vi "GeoData.vi"() -> ()   [LabVIEW 2017] (continued)
H1\n95924\t6057\tCedar ridge\tCA\tNevada County\tH1\n95728\t6057\tSoda springs\tCA\tNevada County\tH1\n95602\t6057\tAuburn\tCA\tNevada County\tH1\n95986\t6057\tWashington\tCA\tNevada County\tH1\n95712\t6057\tChicago park\tCA\tNevada County\tH1\n96161\t6057\tTruckee\tCA\tNevada County\tH1\n95949\t6057\tGrass valley\tCA\tNevada County\tH1\n95975\t6057\tRough and ready\tCA\tNevada County\tH1\n96160\t6057\tTruckee\tCA\tNevada County\tH1\n96111\t6057\tFloriston\tCA\tNevada County\tH1\n95945\t6057\tGrass valley\tCA\tNevada County\tH1\n95960\t6057\tNorth san juan\tCA\tNevada County\tH1\n95959\t6057\tNevada city\tCA\tNevada County\tH1\n90638\t6059\tLa mirada\tCA\tOrange County\tH1\n90680\t6059\tStanton\tCA\tOrange County\tH1\n92623\t6059\tIrvine\tCA\tOrange County\tH1\n92675\t6059\tSan juan capistrano\tCA\tOrange County\tH1\n92662\t6059\tNewport beach\tCA\tOrange County\tH1\n92693\t6059\tSan juan capistrano\tCA\tOrange County\tH1\n92694\t6059\tLadera ranch\tCA\tOrange County\tH1\n92825\t6059\tAnaheim\tCA\tOrange County\tH1\n92870\t6059\tPlacentia\tCA\tOrange County\tH1\n92811\t6059\tAtwood\tCA\tOrange County\tH1\n92616\t6059\tIrvine\tCA\tOrange County\tH1\n92702\t6059\tSanta ana\tCA\tOrange County\tH1\n92602\t6059\tIrvine\tCA\tOrange County\tH1\n92617\t6059\tIrvine\tCA\tOrange County\tH1\n92627\t6059\tCosta mesa\tCA\tOrange County\tH1\n92651\t6059\tLaguna beach\tCA\tOrange County\tH1\n92661\t6059\tNewport beach\tCA\tOrange County\tH1\n92637\t6059\tLaguna woods\tCA\tOrange County\tH1\n92688\t6059\tRancho santa margarita\tCA\tOrange County\tH1\n92654\t6059\tLaguna hills\tCA\tOrange County\tH1\n92782\t6059\tTustin\tCA\tOrange County\tH1\n92861\t6059\tVilla park\tCA\tOrange County\tH1\n92867\t6059\tOrange\tCA\tOrange County\tH1\n92886\t6059\tYorba linda\tCA\tOrange County\tH1\n92655\t6059\tMidway city\tCA\tOrange County\tH1\n92678\t6059\tTrabuco canyon\tCA\tOrange County\tH1\n90720\t6059\tLos alamitos\tCA\tOrange County\tH1\n90622\t6059\tBuena park\tCA\tOrange County\tH1\n92609\t6059\tEl toro\tCA\tOrange County\tH1\n92672\t6059\tSan clemente\tCA\tOrange County\tH1\n92630\t6059\tLake forest\tCA\tOrange County\tH1\n92648\t6059\tHuntington beach\tCA\tOrange County\tH1\n92692\t6059\tMission viejo\tCA\tOrange County\tH1\n92701\t6059\tSanta ana\tCA\tOrange County\tH1\n92801\t6059\tAnaheim\tCA\tOrange County\tH1\n92804\t6059\tAnaheim\tCA\tOrange County\tH1\n92808\t6059\tAnaheim\tCA\tOrange County\tH1\n92821\t6059\tBrea\tCA\tOrange County\tH1\n92831\t6059\tFullerton\tCA\tOrange County\tH1\n92840\t6059\tGarden grove\tCA\tOrange County\tH1\n92803\t6059\tAnaheim\tCA\tOrange County\tH1\n92868\t6059\tOrange\tCA\tOrange County\tH1\n92822\t6059\tBrea\tCA\tOrange County\tH1\n92863\t6059\tOrange\tCA\tOrange County\tH1\n90721\t6059\tLos alamitos\tCA\tOrange County\tH1\n92846\t6059\tGarden grove\tCA\tOrange County\tH1\n92698\t6059\tAliso viejo\tCA\tOrange County\tH1\n92864\t6059\tOrange\tCA\tOrange County\tH1\n90624\t6059\tBuena park\tCA\tOrange County\tH1\n90740\t6059\tSeal beach\tCA\tOrange County\tH1\n90621\t6059\tBuena park\tCA\tOrange County\tH1\n90620\t6059\tBuena park\tCA\tOrange County\tH1\n92603\t6059\tIrvine\tCA\tOrange County\tH1\n92649\t6059\tHuntington beach\tCA\tOrange County\tH1\n92663\t6059\tNewport beach\tCA\tOrange County\tH1\n92657\t6059\tNewport coast\tCA\tOrange County\tH1\n92677\t6059\tLaguna niguel\tCA\tOrange County\tH1\n92691\t6059\tMission viejo\tCA\tOrange County\tH1\n92780\t6059\tTustin\tCA\tOrange County\tH1\n92805\t6059\tAnaheim\tCA\tOrange County\tH1\n92807\t6059\tAnaheim\tCA\tOrange County\tH1\n92704\t6059\tSanta ana\tCA\tOrange County\tH1\n92706\t6059\tSanta ana\tCA\tOrange County\tH1\n92806\t6059\tAnaheim\tCA\tOrange County\tH1\n92841\t6059\tGarden grove\tCA\tOrange County\tH1\n92843\t6059\tGarden grove\tCA\tOrange County\tH1\n92711\t6059\tSanta ana\tCA\tOrange County\tH1\n92815\t6059\tAnaheim\tCA\tOrange County\tH1\n92869\t6059\tOrange\tCA\tOrange County\tH1\n90633\t6059\tLa habra\tCA\tOrange County\tH1\n90742\t6059\tSunset beach\tCA\tOrange County\tH1\n92857\t6059\tOrange\tCA\tOrange County\tH1\n90743\t6059\tSurfside\tCA\tOrange County\tH1\n90815\t6059\tLong beach\tCA\tOrange County\tH1\n92604\t6059\tIrvine\tCA\tOrange County\tH1\n92612\t6059\tIrvine\tCA\tOrange County\tH1\n92618\t6059\tIrvine\tCA\tOrange County\tH1\n92620\t6059\tIrvine\tCA\tOrange County\tH1\n92625\t6059\tCorona del mar\tCA\tOrange County\tH1\n92614\t6059\tIrvine\tCA\tOrange County\tH1\n92629\t6059\tDana point\tCA\tOrange County\tH1\n92697\t6059\tIrvine\tCA\tOrange County\tH1\n92802\t6059\tAnaheim\tCA\tOrange County\tH1\n92823\t6059\tBrea\tCA\tOrange County\tH1\n92844\t6059\tGarden grove\tCA\tOrange County\tH1\n92866\t6059\tOrange\tCA\tOrange County\tH1\n92619\t6059\tIrvine\tCA\tOrange County\tH1\n92676\t6059\tSilverado\tCA\tOrange County\tH1\n92684\t6059\tWestminster\tCA\tOrange County\tH1\n92871\t6059\tPlacentia\tCA\tOrange County\tH1\n92816\t6059\tAnaheim\tCA\tOrange County\tH1\n90631\t6059\tLa habra\tCA\tOrange County\tH1\n92610\t6059\tFoothill ranch\tCA\tOrange County\tH1\n92626\t6059\tCosta mesa\tCA\tOrange County\tH1\n92624\t6059\tCapistrano beach\tCA\tOrange County\tH1\n92647\t6059\tHuntington beach\tCA\tOrange County\tH1\n92673\t6059\tSan clemente\tCA\tOrange County\tH1\n92685\t6059\tWestminster\tCA\tOrange County\tH1\n92707\t6059\tSanta ana\tCA\tOrange County\tH1\n92708\t6059\tFountain valley\tCA\tOrange County\tH1\n92781\t6059\tTustin\tCA\tOrange County\tH1\n92812\t6059\tAnaheim\tCA\tOrange County\tH1\n92865\t6059\tOrange\tCA\tOrange County\tH1\n92887\t6059\tYorba linda\tCA\tOrange County\tH1\n92817\t6059\tAnaheim\tCA\tOrange County\tH1\n92834\t6059\tFullerton\tCA\tOrange County\tH1\n92838\t6059\tFullerton\tCA\tOrange County\tH1\n92607\t6059\tLaguna niguel\tCA\tOrange County\tH1\n92859\t6059\tOrange\tCA\tOrange County\tH1\n90632\t6059\tLa habra\tCA\tOrange County\tH1\n92836\t6059\tFullerton\tCA\tOrange County\tH1\n90623\t6059\tLa palma\tCA\tOrange County\tH1\n92653\t6059\tLaguna hills\tCA\tOrange County\tH1\n92646\t6059\tHuntington beach\tCA\tOrange County\tH1\n92650\t6059\tEast irvine\tCA\tOrange County\tH1\n92679\t6059\tTrabuco canyon\tCA\tOrange County\tH1\n92703\t6059\tSanta ana\tCA\tOrange County\tH1\n92705\t6059\tSanta ana\tCA\tOrange County\tH1\n92845\t6059\tGarden grove\tCA\tOrange County\tH1\n92837\t6059\tFullerton\tCA\tOrange County\tH1\n92832\t6059\tFullerton\tCA\tOrange County\tH1\n92652\t6059\tLaguna beach\tCA\tOrange County\tH1\n92799\t6059\tSanta ana\tCA\tOrange County\tH1\n92728\t6059\tFountain valley\tCA\tOrange County\tH1\n92735\t6059\tSanta ana\tCA\tOrange County\tH1\n92814\t6059\tAnaheim\tCA\tOrange County\tH1\n92862\t6059\tOrange\tCA\tOrange County\tH1\n90808\t6059\tLong beach\tCA\tOrange County\tH1\n90630\t6059\tCypress\tCA\tOrange County\tH1\n92605\t6059\tHuntington beach\tCA\tOrange County\tH1\n92606\t6059\tIrvine\tCA\tOrange County\tH1\n92656\t6059\tAliso viejo\tCA\tOrange County\tH1\n92660\t6059\tNewport beach\tCA\tOrange County\tH1\n92674\t6059\tSan clemente\tCA\tOrange County\tH1\n92683\t6059\tWestminster\tCA\tOrange County\tH1\n92658\t6059\tNewport beach\tCA\tOrange County\tH1\n92690\t6059\tMission viejo\tCA\tOrange County\tH1\n92628\t6059\tCosta mesa\tCA\tOrange County\tH1\n92835\t6059\tFullerton\tCA\tOrange County\tH1\n92842\t6059\tGarden grove\tCA\tOrange County\tH1\n92856\t6059\tOrange\tCA\tOrange County\tH1\n92833\t6059\tFullerton\tCA\tOrange County\tH1\n92809\t6059\tAnaheim\tCA\tOrange County\tH1\n92615\t6059\tHuntington beach\tCA\tOrange County\tH1\n92659\t6059\tNewport beach\tCA\tOrange County\tH1\n92885\t6059\tYorba linda\tCA\tOrange County\tH1\n92899\t6059\tAnaheim\tCA\tOrange County\tH1\n95631\t6061\tForesthill\tCA\tPlacer County\tH1\n95722\t6061\tMeadow vista\tCA\tPlacer County\tH1\n95650\t6061\tLoomis\tCA\tPlacer County\tH1\n95661\t6061\tRoseville\tCA\tPlacer County\tH1\n95765\t6061\tRocklin\tCA\tPlacer County\tH1\n96146\t6061\tOlympic valley\tCA\tPlacer County\tH1\n96145\t6061\tTahoe city\tCA\tPlacer County\tH1\n96148\t6061\tTahoe vista\tCA\tPlacer County\tH1\n95701\t6061\tAlta\tCA\tPlacer County\tH1\n95703\t6061\tApplegate\tCA\tPlacer County\tH1\n96141\t6061\tHomewood\tCA\tPlacer County\tH1\n95602\t6061\tAuburn\tCA\tPlacer County\tH1\n95663\t6061\tPenryn\tCA\tPlacer County\tH1\n96143\t6061\tKings beach\tCA\tPlacer County\tH1\n96161\t6061\tTruckee\tCA\tPlacer County\tH1\n95648\t6061\tLincoln\tCA\tPlacer County\tH1\n95626\t6061\tElverta\tCA\tPlacer County\tH1\n95658\t6061\tNewcastle\tCA\tPlacer County\tH1\n95746\t6061\tGranite bay\tCA\tPlacer County\tH1\n95747\t6061\tRoseville\tCA\tPlacer County\tH1\n95713\t6061\tColfax\tCA\tPlacer County\tH1\n95714\t6061\tDutch flat\tCA\tPlacer County\tH1\n95715\t6061\tEmigrant gap\tCA\tPlacer County\tH1\n95717\t6061\tGold run\tCA\tPlacer County\tH1\n95681\t6061\tSheridan\tCA\tPlacer County\tH1\n95610\t6061\tCitrus heights\tCA\tPlacer County\tH1\n95603\t6061\tAuburn\tCA\tPlacer County\tH1\n95604\t6061\tAuburn\tCA\tPlacer County\tH1\n95678\t6061\tRoseville\tCA\tPlacer County\tH1\n95677\t6061\tRocklin\tCA\tPlacer County\tH1\n96142\t6061\tTahoma\tCA\tPlacer County\tH1\n95668\t6061\tPleasant grove\tCA\tPlacer County\tH1\n96140\t6061\tCarnelian bay\tCA\tPlacer County\tH1\n95736\t6061\tWeimar\tCA\tPlacer County\tH1\n95983\t6063\tTaylorsville\tCA\tPlumas County\tH1\n96105\t6063\tChilcoot\tCA\tPlumas County\tH1\n96122\t6063\tPortola\tCA\tPlumas County\tH1\n95971\t6063\tQuincy\tCA\tPlumas County\tH1\n96135\t6063\tVinton\tCA\tPlumas County\tH1\n95956\t6063\tMeadow valley\tCA\tPlumas County\tH1\n95947\t6063\tGreenville\tCA\tPlumas County\tH1\n95980\t6063\tStorrie\tCA\tPlumas County\tH1\n95915\t6063\tBelden\tCA\tPlumas County\tH1\n95981\t6063\tStrawberry valley\tCA\tPlumas County\tH1\n95930\t6063\tClipper mills\tCA\tPlumas County\tH1\n95984\t6063\tTwain\tCA\tPlumas County\tH1\n96020\t6063\tChester\tCA\tPlumas County\tH1\n96137\t6063\tWestwood\tCA\tPlumas County\tH1\n96129\t6063\tBeckwourth\tCA\tPlumas County\tH1\n95934\t6063\tCrescent mills\tCA\tPlumas County\tH1\n96106\t6063\tClio\tCA\tPlumas County\tH1\n95923\t6063\tCanyon dam\tCA\tPlumas County\tH1\n96103\t6063\tBlairsden graeagle\tCA\tPlumas County\tH1\n92373\t6065\tRedlands\tCA\tRiverside County\tH1\n92595\t6065\tWildomar\tCA\tRiverside County\tH1\n92518\t6065\tMarch air reserve base\tCA\tRiverside County\tH1\n92530\t6065\tLake elsinore\tCA\tRiverside County\tH1\n92548\t6065\tHomeland\tCA\tRiverside County\tH1\n92508\t6065\tRiverside\tCA\tRiverside County\tH1\n92552\t6065\tMoreno valley\tCA\tRiverside County\tH1\n92262\t6065\tPalm springs\tCA\tRiverside County\tH1\n92522\t6065\tRiverside\tCA\tRiverside County\tH1\n92220\t6065\tBanning\tCA\tRiverside County\tH1\n92591\t6065\tTemecula\tCA\tRiverside County\tH1\n92582\t6065\tSan jacinto\tCA\tRiverside County\tH1\n92531\t6065\tLake elsinore\tCA\tRiverside County\tH1\n92562\t6065\tMurrieta\tCA\tRiverside County\tH1\n92551\t6065\tMoreno valley\tCA\tRiverside County\tH1\n92581\t6065\tSan jacinto\tCA\tRiverside County\tH1\n92203\t6065\tIndio\tCA\tRiverside County\tH1\n92211\t6065\tPalm desert\tCA\tRiverside County\tH1\n92590\t6065\tTemecula\tCA\tRiverside County\tH1\n92592\t6065\tTemecula\tCA\tRiverside County\tH1\n92571\t6065\tPerris\tCA\tRiverside County\tH1\n92507\t6065\tRiverside\tCA\tRiverside County\tH1\n92532\t6065\tLake elsinore\tCA\tRiverside County\tH1\n92539\t6065\tAnza\tCA\tRiverside County\tH1\n92563\t6065\tMurrieta\tCA\tRiverside County\tH1\n92567\t6065\tNuevo\tCA\tRiverside County\tH1\n92240\t6065\tDesert hot springs\tCA\tRiverside County\tH1\n92234\t6065\tCathedral city\tCA\tRiverside County\tH1\n92241\t6065\tDesert hot springs\tCA\tRiverside County\tH1\n92883\t6065\tCorona\tCA\tRiverside County\tH1\n92513\t6065\tRiverside\tCA\tRiverside County\tH1\n92248\t6065\tLa quinta\tCA\tRiverside County\tH1\n92517\t6065\tRiverside\tCA\tRiverside County\tH1\n92226\t6065\tBlythe\tCA\tRiverside County\tH1\n92564\t6065\tMurrieta\tCA\tRiverside County\tH1\n92399\t6065\tYucaipa\tCA\tRiverside County\tH1\n92596\t6065\tWinchester\tCA\tRiverside County\tH1\n92586\t6065\tMenifee\tCA\tRiverside County\tH1\n91708\t6065\tChino\tCA\tRiverside County\tH1\n92509\t6065\tJurupa valley\tCA\tRiverside County\tH1\n92519\t6065\tRiverside\tCA\tRiverside County\tH1\n92505\t6065\tRiverside\tCA\tRiverside County\tH1\n92553\t6065\tMoreno valley\tCA\tRiverside County\tH1\n92253\t6065\tLa quinta\tCA\tRiverside County\tH1\n92236\t6065\tCoachella\tCA\tRiverside County\tH1\n92282\t6065\tWhitewater\tCA\tRiverside County\tH1\n92860\t6065\tNorco\tCA\tRiverside County\tH1\n92882\t6065\tCorona\tCA\tRiverside County\tH1\n92514\t6065\tRiverside\tCA\tRiverside County\tH1\n92247\t6065\tLa quinta\tCA\tRiverside County\tH1\n92028\t6065\tFallbrook\tCA\tRiverside County\tH1\n92201\t6065\tIndio\tCA\tRiverside County\tH1\n92585\t6065\tMenifee\tCA\tRiverside County\tH1\n92593\t6065\tTemecula\tCA\tRiverside County\tH1\n91752\t6065\tMira loma\tCA\tRiverside County\tH1\n92555\t6065\tMoreno valley\tCA\tRiverside County\tH1\n92546\t6065\tHemet\tCA\tRiverside County\tH1\n92223\t6065\tBeaumont\tCA\tRiverside County\tH1\n92254\t6065\tMecca\tCA\tRiverside County\tH1\n92230\t6065\tCabazon\tCA\tRiverside County\tH1\n92263\t6065\tPalm springs\tCA\tRiverside County\tH1\n92255\t6065\tPalm desert\tCA\tRiverside County\tH1\n92589\t6065\tTemecula\tCA\tRiverside County\tH1\n92239\t6065\tDesert center\tCA\tRiverside County\tH1\n92210\t6065\tIndian wells\tCA\tRiverside County\tH1\n92320\t6065\tCalimesa\tCA\tRiverside County\tH1\n92584\t6065\tMenifee\tCA\tRiverside County\tH1\n92587\t6065\tMenifee\tCA\tRiverside County\tH1\n92544\t6065\tHemet\tCA\tRiverside County\tH1\n92543\t6065\tHemet\tCA\tRiverside County\tH1\n92503\t6065\tRiverside\tCA\tRiverside County\tH1\n92261\t6065\tPalm desert\tCA\tRiverside County\tH1\n92274\t6065\tThermal\tCA\tRiverside County\tH1\n92202\t6065\tIndio\tCA\tRiverside County\tH1\n92556\t6065\tMoreno valley\tCA\tRiverside County\tH1\n92549\t6065\tIdyllwild\tCA\tRiverside County\tH1\n92258\t6065\tNorth palm springs\tCA\tRiverside County\tH1\n92521\t6065\tRiverside\tCA\tRiverside County\tH1\n92599\t6065\tPerris\tCA\tRiverside County\tH1\n92572\t6065\tPerris\tCA\tRiverside County\tH1\n91762\t6065\tOntario\tCA\tRiverside County\tH1\n92506\t6065\tRiverside\tCA\tRiverside County\tH1\n92504\t6065\tRiverside\tCA\tRiverside County\tH1\n92545\t6065\tHemet\tCA\tRiverside County\tH1\n92536\t6065\tAguanga\tCA\tRiverside County\tH1\n92561\t6065\tMountain center\tCA\tRiverside County\tH1\n92260\t6065\tPalm desert\tCA\tRiverside County\tH1\n92225\t6065\tBlythe\tCA\tRiverside County\tH1\n92270\t6065\tRancho mirage\tCA\tRiverside County\tH1\n92878\t6065\tCorona\tCA\tRiverside County\tH1\n92877\t6065\tCorona\tCA\tRiverside County\tH1\n92502\t6065\tRiverside\tCA\tRiverside County\tH1\n92324\t6065\tColton\tCA\tRiverside County\tH1\n92570\t6065\tPerris\tCA\tRiverside County\tH1\n92583\t6065\tSan jacinto\tCA\tRiverside County\tH1\n92557\t6065\tMoreno valley\tCA\tRiverside County\tH1\n92501\t6065\tRiverside\tCA\tRiverside County\tH1\n92516\t6065\tRiverside\tCA\tRiverside County\tH1\n92264\t6065\tPalm springs\tCA\tRiverside County\tH1\n92235\t6065\tCathedral city\tCA\tRiverside County\tH1\n92276\t6065\tThousand palms\tCA\tRiverside County\tH1\n92879\t6065\tCorona\tCA\tRiverside County\tH1\n92880\t6065\tCorona\tCA\tRiverside County\tH1\n92881\t6065\tCorona\tCA\tRiverside County\tH1\n95630\t6067\tFolsom\tCA\tSacramento County\tH1\n95683\t6067\tSloughhouse\tCA\tSacramento County\tH1\n95820\t6067\tSacramento\tCA\tSacramento County\tH1\n95864\t6067\tSacramento\tCA\tSacramento County\tH1\n95826\t6067\tSacramento\tCA\tSacramento County\tH1\n95690\t6067\tWalnut grove\tCA\tSacramento County\tH1\n95661\t6067\tRoseville\tCA\tSacramento County\tH1\n95611\t6067\tCitrus heights\tCA\tSacramento County\tH1\n95812\t6067\tSacramento\tCA\tSacramento County\tH1\n95823\t6067\tSacramento\tCA\tSacramento County\tH1\n95835\t6067\tSacramento\tCA\tSacramento County\tH1\n95671\t6067\tRepresa\tCA\tSacramento County\tH1\n95662\t6067\tOrangevale\tCA\tSacramento County\tH1\n95814\t6067\tSacramento\tCA\tSacramento County\tH1\n95818\t6067\tSacramento\tCA\tSacramento County\tH1\n95838\t6067\tSacramento\tCA\tSacramento County\tH1\n95831\t6067\tSacramento\tCA\tSacramento County\tH1\n95833\t6067\tSacramento\tCA\tSacramento County\tH1\n95759\t6067\tElk grove\tCA\tSacramento County\tH1\n95853\t6067\tSacramento\tCA\tSacramento County\tH1\n95628\t6067\tFair oaks\tCA\tSacramento County\tH1\n95621\t6067\tCitrus heights\tCA\tSacramento County\tH1\n95741\t6067\tRancho cordova\tCA\tSacramento County\tH1\n95819\t6067\tSacramento\tCA\tSacramento County\tH1\n95830\t6067\tSacramento\tCA\tSacramento County\tH1\n95840\t6067\tSacramento\tCA\tSacramento County\tH1\n95626\t6067\tElverta\tCA\tSacramento County\tH1\n95673\t6067\tRio linda\tCA\tSacramento County\tH1\n95670\t6067\tRancho cordova\tCA\tSacramento County\tH1\n95652\t6067\tMcclellan\tCA\tSacramento County\tH1\n95660\t6067\tNorth highlands\tCA\tSacramento County\tH1\n95757\t6067\tElk grove\tCA\tSacramento County\tH1\n95815\t6067\tSacramento\tCA\tSacramento County\tH1\n95822\t6067\tSacramento\tCA\tSacramento County\tH1\n95693\t6067\tWilton\tCA\tSacramento County\tH1\n95828\t6067\tSacramento\tCA\tSacramento County\tH1\n95834\t6067\tSacramento\tCA\tSacramento County\tH1\n95860\t6067\tSacramento\tCA\tSacramento County\tH1\n95842\t6067\tSacramento\tCA\tSacramento County\tH1\n95813\t6067\tSacramento\tCA\tSacramento County\tH1\n95867\t6067\tSacramento\tCA\tSacramento County\tH1\n95836\t6067\tSacramento\tCA\tSacramento County\tH1\n94571\t6067\tRio vista\tCA\tSacramento County\tH1\n95624\t6067\tElk grove\tCA\tSacramento County\tH1\n95632\t6067\tGalt\tCA\tSacramento County\tH1\n95825\t6067\tSacramento\tCA\tSacramento County\tH1\n95821\t6067\tSacramento\tCA\tSacramento County\tH1\n95841\t6067\tSacramento\tCA\tSacramento County\tH1\n95827\t6067\tSacramento\tCA\tSacramento County\tH1\n95843\t6067\tAntelope\tCA\tSacramento County\tH1\n95837\t6067\tSacramento\tCA\tSacramento County\tH1\n95866\t6067\tSacramento\tCA\tSacramento County\tH1\n95894\t6067\tSacramento\tCA\tSacramento County\tH1\n95816\t6067\tSacramento\tCA\tSacramento County\tH1\n95824\t6067\tSacramento\tCA\tSacramento County\tH1\n95829\t6067\tSacramento\tCA\tSacramento County\tH1\n95832\t6067\tSacramento\tCA\tSacramento County\tH1\n95638\t6067\tHerald\tCA\tSacramento County\tH1\n95641\t6067\tIsleton\tCA\tSacramento County\tH1\n95851\t6067\tSacramento\tCA\tSacramento County\tH1\n95615\t6067\tCourtland\tCA\tSacramento County\tH1\n95608\t6067\tCarmichael\tCA\tSacramento County\tH1\n95610\t6067\tCitrus heights\tCA\tSacramento County\tH1\n95609\t6067\tCarmichael\tCA\tSacramento County\tH1\n95655\t6067\tMather\tCA\tSacramento County\tH1\n95758\t6067\tElk grove\tCA\tSacramento County\tH1\n95811\t6067\tSacramento\tCA\tSacramento County\tH1\n95678\t6067\tRoseville\tCA\tSacramento County\tH1\n95817\t6067\tSacramento\tCA\tSacramento County\tH1\n95742\t6067\tRancho cordova\tCA\tSacramento County\tH1\n95852\t6067\tSacramento\tCA\tSacramento County\tH1\n95763\t6067\tFolsom\tCA\tSacramento County\tH1\n95865\t6067\tSacramento\tCA\tSacramento County\tH1\n95639\t6067\tHood\tCA\tSacramento County\tH1\n95680\t6067\tRyde\tCA\tSacramento County\tH1\n95004\t6069\tAromas\tCA\tSan Benito County\tH1\n93925\t6069\tChualar\tCA\tSan Benito County\tH1\n95043\t6069\tPaicines\tCA\tSan Benito County\tH1\n95024\t6069\tHollister\tCA\tSan Benito County\tH1\n95075\t6069\tTres pinos\tCA\tSan Benito County\tH1\n95045\t6069\tSan juan bautista\tCA\tSan Benito County\tH1\n95023\t6069\tHollister\tCA\tSan Benito County\tH1\n92344\t6071\tHesperia\tCA\tSan Bernardino County\tH1\n92345\t6071\tHesperia\tCA\tSan Bernardino County\tH1\n92373\t6071\tRedlands\tCA\tSan Bernardino County\tH1\n92356\t6071\tLucerne valley\tCA\tSan Bernardino County\tH1\n92394\t6071\tVictorville\tCA\tSan Bernardino County\tH1\n92335\t6071\tFontana\tCA\tSan Bernardino County\tH1\n92404\t6071\tSan bernardino\tCA\tSan Bernardino County\tH1\n91730\t6071\tRancho cucamonga\tCA\tSan Bernardino County\tH1\n91764\t6071\tOntario\tCA\tSan Bernardino County\tH1\n92372\t6071\tPinon hills\tCA\tSan Bernardino County\tH1\n91785\t6071\tUpland\tCA\tSan Bernardino County\tH1\n92305\t6071\tAngelus oaks\tCA\tSan Bernardino County\tH1\n92317\t6071\tBlue jay\tCA\tSan Bernardino County\tH1\n91759\t6071\tMt baldy\tCA\tSan Bernardino County\tH1\n92352\t6071\tLake arrowhead\tCA\tSan Bernardino County\tH1\n92402\t6071\tSan bernardino\tCA\tSan Bernardino County\tH1\n91784\t6071\tUpland\tCA\tSan Bernardino County\tH1\n91763\t6071\tMontclair\tCA\tSan Bernardino County\tH1\n92423\t6071\tSan bernardino\tCA\tSan Bernardino County\tH1\n92277\t6071\tTwentynine palms\tCA\tSan Bernardino County\tH1\n92284\t6071\tYucca valley\tCA\tSan Bernardino County\tH1\n92285\t6071\tLanders\tCA\tSan Bernardino County\tH1\n92332\t6071\tEssex\tCA\tSan Bernardino County\tH1\n92366\t6071\tMountain pass\tCA\tSan Bernardino County\tH1\n92312\t6071\tBarstow\tCA\tSan Bernardino County\tH1\n92369\t6071\tPatton\tCA\tSan Bernardino County\tH1\n92418\t6071\tSan bernardino\tCA\tSan Bernardino County\tH1\n93555\t6071\tRidgecrest\tCA\tSan Bernardino County\tH1\n92313\t6071\tGrand terrace\tCA\tSan Bernardino County\tH1\n92316\t6071\tBloomington\tCA\tSan Bernardino County\tH1\n92365\t6071\tNewberry springs\tCA\tSan Bernardino County\tH1\n92368\t6071\tOro grande\tCA\tSan Bernardino County\tH1\n92342\t6071\tHelendale\tCA\tSan Bernardino County\tH1\n92406\t6071\tSan bernardino\tCA\tSan Bernardino County\tH1\n91709\t6071\tChino hills\tCA\tSan Bernardino County\tH1\n92364\t6071\tNipton\tCA\tSan Bernardino County\tH1\n92340\t6071\tHesperia\tCA\tSan Bernardino County\tH1\n92315\t6071\tBig bear lake\tCA\tSan Bernardino County\tH1\n92393\t6071\tVictorville\tCA\tSan Bernardino County\tH1\n92382\t6071\tRunning springs\tCA\tSan Bernardino County\tH1\n92304\t6071\tAmboy\tCA\tSan Bernardino County\tH1\n92403\t6071\tSan bernardino\tCA\tSan Bernardino County\tH1\n92318\t6071\tBryn mawr\tCA\tSan Bernardino County\tH1\n92399\t6071\tYucaipa\tCA\tSan Bernardino County\tH1\n91710\t6071\tChino\tCA\tSan Bernardino County\tH1\n91737\t6071\tRancho cucamonga\tCA\tSan Bernardino County\tH1\n91708\t6071\tChino\tCA\tSan Bernardino County\tH1\n92509\t6071\tJurupa valley\tCA\tSan Bernardino County\tH1\n92256\t6071\tMorongo valley\tCA\tSan Bernardino County\tH1\n92386\t6071\tSugarloaf\tCA\tSan Bernardino County\tH1\n92278\t6071\tTwentynine palms\tCA\tSan Bernardino County\tH1\n93562\t6071\tTrona\tCA\tSan Bernardino County\tH1\n92392\t6071\tVictorville\tCA\tSan Bernardino County\tH1\n92374\t6071\tRedlands\tCA\tSan Bernardino County\tH1\n92363\t6071\tNeedles\tCA\tSan Bernardino County\tH1\n92310\t6071\tFort irwin\tCA\tSan Bernardino County\tH1\n92407\t6071\tSan bernardino\tCA\tSan Bernardino County\tH1\n91701\t6071\tRancho cucamonga\tCA\tSan Bernardino County\tH1\n91761\t6071\tOntario\tCA\tSan Bernardino County\tH1\n91729\t6071\tRancho cucamonga\tCA\tSan Bernardino County\tH1\n91752\t6071\tMira loma\tCA\tSan Bernardino County\tH1\n92223\t6071\tBeaumont\tCA\tSan Bernardino County\tH1\n92301\t6071\tAdelanto\tCA\tSan Bernardino County\tH1\n92329\t6071\tPhelan\tCA\tSan Bernardino County\tH1\n92401\t6071\tSan bernardino\tCA\tSan Bernardino County\tH1\n92391\t6071\tTwin peaks\tCA\tSan Bernardino County\tH1\n92350\t6071\tLoma linda\tCA\tSan Bernardino County\tH1\n92331\t6071\tFontana\tCA\tSan Bernardino County\tH1\n92280\t6071\tVidal\tCA\tSan Bernardino County\tH1\n92322\t6071\tCedarpines park\tCA\tSan Bernardino County\tH1\n92341\t6071\tGreen valley lake\tCA\tSan Bernardino County\tH1\n92267\t6071\tParker dam\tCA\tSan Bernardino County\tH1\n93516\t6071\tBoron\tCA\tSan Bernardino County\tH1\n92336\t6071\tFontana\tCA\tSan Bernardino County\tH1\n92346\t6071\tHighland\tCA\tSan Bernardino County\tH1\n92359\t6071\tMentone\tCA\tSan Bernardino County\tH1\n92371\t6071\tPhelan\tCA\tSan Bernardino County\tH1\n92311\t6071\tBarstow\tCA\tSan Bernardino County\tH1\n92377\t6071\tRialto\tCA\tSan Bernardino County\tH1\n92395\t6071\tVictorville\tCA\tSan Bernardino County\tH1\n92397\t6071\tWrightwood\tCA\tSan Bernardino County\tH1\n92314\t6071\tBig bear city\tCA\tSan Bernardino County\tH1\n92320\t6071\tCalimesa\tCA\tSan Bernardino County\tH1\n91786\t6071\tUpland\tCA\tSan Bernardino County\tH1\n92411\t6071\tSan bernardino\tCA\tSan Bernardino County\tH1\n92309\t6071\tBaker\tCA\tSan Bernardino County\tH1\n92385\t6071\tSkyforest\tCA\tSan Bernardino County\tH1\n92378\t6071\tRimforest\tCA\tSan Bernardino County\tH1\n92358\t6071\tLytle creek\tCA\tSan Bernardino County\tH1\n92376\t6071\tRialto\tCA\tSan Bernardino County\tH1\n92325\t6071\tCrestline\tCA\tSan Bernardino County\tH1\n91739\t6071\tRancho cucamonga\tCA\tSan Bernardino County\tH1\n91762\t6071\tOntario\tCA\tSan Bernardino County\tH1\n91766\t6071\tPomona\tCA\tSan Bernardino County\tH1\n92410\t6071\tSan bernardino\tCA\tSan Bernardino County\tH1\n92225\t6071\tBlythe\tCA\tSan Bernardino County\tH1\n92252\t6071\tJoshua tree\tCA\tSan Bernardino County\tH1\n92308\t6071\tApple valley\tCA\tSan Bernardino County\tH1\n92375\t6071\tRedlands\tCA\tSan Bernardino County\tH1\n92242\t6071\tEarp\tCA\tSan Bernardino County\tH1\n92339\t6071\tForest falls\tCA\tSan Bernardino County\tH1\n92338\t6071\tLudlow\tCA\tSan Bernardino County\tH1\n92321\t6071\tCedar glen\tCA\tSan Bernardino County\tH1\n92268\t6071\tPioneertown\tCA\tSan Bernardino County\tH1\n92324\t6071\tColton\tCA\tSan Bernardino County\tH1\n92405\t6071\tSan bernardino\tCA\tSan Bernardino County\tH1\n92354\t6071\tLoma linda\tCA\tSan Bernardino County\tH1\n92337\t6071\tFontana\tCA\tSan Bernardino County\tH1\n92347\t6071\tHinkley\tCA\tSan Bernardino County\tH1\n92408\t6071\tSan bernardino\tCA\tSan Bernardino County\tH1\n92413\t6071\tSan bernardino\tCA\tSan Bernardino County\tH1\n92427\t6071\tSan bernardino\tCA\tSan Bernardino County\tH1\n92307\t6071\tApple valley\tCA\tSan Bernardino County\tH1\n92880\t6071\tCorona\tCA\tSan Bernardino County\tH1\n92333\t6071\tFawnskin\tCA\tSan Bernardino County\tH1\n92327\t6071\tDaggett\tCA\tSan Bernardino County\tH1\n92334\t6071\tFontana\tCA\tSan Bernardino County\tH1\n92286\t6071\tYucca valley\tCA\tSan Bernardino County\tH1\n92415\t6071\tSan bernardino\tCA\tSan Bernardino County\tH1\n91743\t6071\tGuasti\tCA\tSan Bernardino County\tH1\n92398\t6071\tYermo\tCA\tSan Bernardino County\tH1\n92323\t6071\tCima\tCA\tSan Bernardino County\tH1\n92357\t6071\tLoma linda\tCA\tSan Bernardino County\tH1\n91901\t6073\tAlpine\tCA\tSan Diego County\tH1\n91950\t6073\tNational city\tCA\tSan Diego County\tH1\n91945\t6073\tLemon grove\tCA\tSan Diego County\tH1\n92036\t6073\tJulian\tCA\tSan Diego County\tH1\n92037\t6073\tLa jolla\tCA\tSan Diego County\tH1\n92109\t6073\tSan diego\tCA\tSan Diego County\tH1\n92111\t6073\tSan diego\tCA\tSan Diego County\tH1\n92093\t6073\tLa jolla\tCA\tSan Diego County\tH1\n92120\t6073\tSan diego\tCA\tSan Diego County\tH1\n92119\t6073\tSan diego\tCA\tSan Diego County\tH1\n92169\t6073\tSan diego\tCA\tSan Diego County\tH1\n92192\t6073\tSan diego\tCA\tSan Diego County\tH1\n92030\t6073\tEscondido\tCA\tSan Diego County\tH1\n92066\t6073\tRanchita\tCA\tSan Diego County\tH1\n92153\t6073\tSan diego\tCA\tSan Diego County\tH1\n92166\t6073\tSan diego\tCA\tSan Diego County\tH1\n92136\t6073\tSan diego\tCA\tSan Diego County\tH1\n91946\t6073\tLemon grove\tCA\tSan Diego County\tH1\n92013\t6073\tCarlsbad\tCA\tSan Diego County\tH1\n92175\t6073\tSan diego\tCA\tSan Diego County\tH1\n92191\t6073\tSan diego\tCA\tSan Diego County\tH1\n91931\t6073\tGuatay\tCA\tSan Diego County\tH1\n92199\t6073\tSan diego\tCA\tSan Diego County\tH1\n91911\t6073\tChula vista\tCA\tSan Diego County\tH1\n92004\t6073\tBorrego springs\tCA\tSan Diego County\tH1\n92020\t6073\tEl cajon\tCA\tSan Diego County\tH1\n91941\t6073\tLa mesa\tCA\tSan Diego County\tH1\n91943\t6073\tLa mesa\tCA\tSan Diego County\tH1\n92007\t6073\tCardiff by the sea\tCA\tSan Diego County\tH1\n92102\t6073\tSan diego\tCA\tSan Diego County\tH1\n92064\t6073\tPoway\tCA\tSan Diego County\tH1\n92061\t6073\tPauma valley\tCA\tSan Diego County\tH1\n92116\t6073\tSan diego\tCA\tSan Diego County\tH1\n92196\t6073\tSan diego\tCA\tSan Diego County\tH1\n92132\t6073\tSan diego\tCA\tSan Diego County\tH1\n91963\t6073\tPotrero\tCA\tSan Diego County\tH1\n92051\t6073\tOceanside\tCA\tSan Diego County\tH1\n92052\t6073\tOceanside\tCA\tSan Diego County\tH1\n92055\t6073\tCamp pendleton\tCA\tSan Diego County\tH1\n92158\t6073\tSan diego\tCA\tSan Diego County\tH1\n92179\t6073\tSan diego\tCA\tSan Diego County\tH1\n92197\t6073\tSan diego\tCA\tSan Diego County\tH1\n92022\t6073\tEl cajon\tCA\tSan Diego County\tH1\n92023\t6073\tEncinitas\tCA\tSan Diego County\tH1\n91932\t6073\tImperial beach\tCA\tSan Diego County\tH1\n92018\t6073\tCarlsbad\tCA\tSan Diego County\tH1\n92027\t6073\tEscondido\tCA\tSan Diego County\tH1\n91914\t6073\tChula vista\tCA\tSan Diego County\tH1\n91978\t6073\tSpring valley\tCA\tSan Diego County\tH1\n92105\t6073\tSan diego\tCA\tSan Diego County\tH1\n92108\t6073\tSan diego\tCA\tSan Diego County\tH1\n92058\t6073\tOceanside\tCA\tSan Diego County\tH1\n92085\t6073\tVista\tCA\tSan Diego County\tH1\n92114\t6073\tSan diego\tCA\tSan Diego County\tH1\n92173\t6073\tSan ysidro\tCA\tSan Diego County\tH1\n92176\t6073\tSan diego\tCA\tSan Diego County\tH1\n92592\t6073\tTemecula\tCA\tSan Diego County\tH1\n92672\t6073\tSan clemente\tCA\tSan Diego County\tH1\n92039\t6073\tLa jolla\tCA\tSan Diego County\tH1\n92134\t6073\tSan diego\tCA\tSan Diego County\tH1\n92060\t6073\tPalomar mountain\tCA\tSan Diego County\tH1\n91910\t6073\tChula vista\tCA\tSan Diego County\tH1\n92008\t6073\tCarlsbad\tCA\tSan Diego County\tH1\n92011\t6073\tCarlsbad\tCA\tSan Diego County\tH1\n92014\t6073\tDel mar\tCA\tSan Diego County\tH1\n92024\t6073\tEncinitas\tCA\tSan Diego County\tH1\n91977\t6073\tSpring valley\tCA\tSan Diego County\tH1\n92009\t6073\tCarlsbad\tCA\tSan Diego County\tH1\n92101\t6073\tSan diego\tCA\tSan Diego County\tH1\n92069\t6073\tSan marcos\tCA\tSan Diego County\tH1\n92081\t6073\tVista\tCA\tSan Diego County\tH1\n92067\t6073\tRancho santa fe\tCA\tSan Diego County\tH1\n92110\t6073\tSan diego\tCA\tSan Diego County\tH1\n92138\t6073\tSan diego\tCA\tSan Diego County\tH1\n92113\t6073\tSan diego\tCA\tSan Diego County\tH1\n92126\t6073\tSan diego\tCA\tSan Diego County\tH1\n92130\t6073\tSan diego\tCA\tSan Diego County\tH1\n92117\t6073\tSan diego\tCA\tSan Diego County\tH1\n92127\t6073\tSan diego\tCA\tSan Diego County\tH1\n92152\t6073\tSan diego\tCA\tSan Diego County\tH1\n92195\t6073\tSan diego\tCA\tSan Diego County\tH1\n92072\t6073\tSantee\tCA\tSan Diego County\tH1\n92159\t6073\tSan diego\tCA\tSan Diego County\tH1\n92174\t6073\tSan diego\tCA\tSan Diego County\tH1\n92046\t6073\tEscondido\tCA\tSan Diego County\tH1\n92142\t6073\tSan diego\tCA\tSan Diego County\tH1\n92074\t6073\tPoway\tCA\tSan Diego County\tH1\n92049\t6073\tOceanside\tCA\tSan Diego County\tH1\n92068\t6073\tSan luis rey\tCA\tSan Diego County\tH1\n91917\t6073\tDulzura\tCA\tSan Diego County\tH1\n92096\t6073\tSan marcos\tCA\tSan Diego County\tH1\n91908\t6073\tBonita\tCA\tSan Diego County\tH1\n91915\t6073\tChula vista\tCA\tSan Diego County\tH1\n92028\t6073\tFallbrook\tCA\tSan Diego County\tH1\n92029\t6073\tEscondido\tCA\tSan Diego County\tH1\n92054\t6073\tOceanside\tCA\tSan Diego County\tH1\n91951\t6073\tNational city\tCA\tSan Diego County\tH1\n91916\t6073\tDescanso\tCA\tSan Diego County\tH1\n91962\t6073\tPine valley\tCA\tSan Diego County\tH1\n91976\t6073\tSpring valley\tCA\tSan Diego County\tH1\n92103\t6073\tSan diego\tCA\tSan Diego County\tH1\n92131\t6073\tSan diego\tCA\tSan Diego County\tH1\n92079\t6073\tSan marcos\tCA\tSan Diego County\tH1\n92143\t6073\tSan ysidro\tCA\tSan Diego County\tH1\n92170\t6073\tSan diego\tCA\tSan Diego County\tH1\n92171\t6073\tSan diego\tCA\tSan Diego County\tH1\n92168\t6073\tSan diego\tCA\tSan Diego County\tH1\n91980\t6073\tTecate\tCA\tSan Diego County\tH1\n92165\t6073\tSan diego\tCA\tSan Diego County\tH1\n92160\t6073\tSan diego\tCA\tSan Diego County\tH1\n91906\t6073\tCampo\tCA\tSan Diego County\tH1\n91942\t6073\tLa mesa\tCA\tSan Diego County\tH1\n92040\t6073\tLakeside\tCA\tSan Diego County\tH1\n91934\t6073\tJacumba\tCA\tSan Diego County\tH1\n92083\t6073\tVista\tCA\tSan Diego County\tH1\n92084\t6073\tVista\tCA\tSan Diego County\tH1\n92104\t6073\tSan diego\tCA\tSan Diego County\tH1\n92065\t6073\tRamona\tCA\tSan Diego County\tH1\n92059\t6073\tPala\tCA\tSan Diego County\tH1\n92086\t6073\tWarner springs\tCA\tSan Diego County\tH1\n92122\t6073\tSan diego\tCA\tSan Diego County\tH1\n92123\t6073\tSan diego\tCA\tSan Diego County\tH1\n92115\t6073\tSan diego\tCA\tSan Diego County\tH1\n92150\t6073\tSan diego\tCA\tSan Diego County\tH1\n92163\t6073\tSan diego\tCA\tSan Diego County\tH1\n91912\t6073\tChula vista\tCA\tSan Diego County\tH1\n91944\t6073\tLa mesa\tCA\tSan Diego County\tH1\n92137\t6073\tSan diego\tCA\tSan Diego County\tH1\n92167\t6073\tSan diego\tCA\tSan Diego County\tH1\n91903\t6073\tAlpine\tCA\tSan Diego County\tH1\n91902\t6073\tBonita\tCA\tSan Diego County\tH1\n92021\t6073\tEl cajon\tCA\tSan Diego County\tH1\n92025\t6073\tEscondido\tCA\tSan Diego County\tH1\n92010\t6073\tCarlsbad\tCA\tSan Diego County\tH1\n92019\t6073\tEl cajon\tCA\tSan Diego County\tH1\n92003\t6073\tBonsall\tCA\tSan Diego County\tH1\n92071\t6073\tSantee\tCA\tSan Diego County\tH1\n92056\t6073\tOceanside\tCA\tSan Diego County\tH1\n92075\t6073\tSolana beach\tCA\tSan Diego County\tH1\n92078\t6073\tSan marcos\tCA\tSan Diego County\tH1\n92088\t6073\tFallbrook\tCA\tSan Diego County\tH1\n92107\t6073\tSan diego\tCA\tSan Diego County\tH1\n92070\t6073\tSanta ysabel\tCA\tSan Diego County\tH1\n92121\t6073\tSan diego\tCA\tSan Diego County\tH1\n92124\t6073\tSan diego\tCA\tSan Diego County\tH1\n92128\t6073\tSan diego\tCA\tSan Diego County\tH1\n92129\t6073\tSan diego\tCA\tSan Diego County\tH1\n92118\t6073\tCoronado\tCA\tSan Diego County\tH1\n92154\t6073\tSan diego\tCA\tSan Diego County\tH1\n92172\t6073\tSan diego\tCA\tSan Diego County\tH1\n92536\t6073\tAguanga\tCA\tSan Diego County\tH1\n92112\t6073\tSan diego\tCA\tSan Diego County\tH1\n91905\t6073\tBoulevard\tCA\tSan Diego County\tH1\n92178\t6073\tCoronado\tCA\tSan Diego County\tH1\n92147\t6073\tSan diego\tCA\tSan Diego County\tH1\n92193\t6073\tSan diego\tCA\tSan Diego County\tH1\n92155\t6073\tSan diego\tCA\tSan Diego County\tH1\n92145\t6073\tSan diego\tCA\tSan Diego County\tH1\n92135\t6073\tSan diego\tCA\tSan Diego County\tH1\n91913\t6073\tChula vista\tCA\tSan Diego County\tH1\n92026\t6073\tEscondido\tCA\tSan Diego County\tH1\n91933\t6073\tImperial beach\tCA\tSan Diego County\tH1\n92033\t6073\tEscondido\tCA\tSan Diego County\tH1\n91921\t6073\tChula vista\tCA\tSan Diego County\tH1\n92038\t6073\tLa jolla\tCA\tSan Diego County\tH1\n91935\t6073\tJamul\tCA\tSan Diego County\tH1\n92082\t6073\tValley center\tCA\tSan Diego County\tH1\n92091\t6073\tRancho santa fe\tCA\tSan Diego County\tH1\n92057\t6073\tOceanside\tCA\tSan Diego County\tH1\n92106\t6073\tSan diego\tCA\tSan Diego County\tH1\n92139\t6073\tSan diego\tCA\tSan Diego County\tH1\n92140\t6073\tSan diego\tCA\tSan Diego County\tH1\n92198\t6073\tSan diego\tCA\tSan Diego County\tH1\n92177\t6073\tSan diego\tCA\tSan Diego County\tH1\n91979\t6073\tSpring valley\tCA\tSan Diego County\tH1\n92149\t6073\tSan diego\tCA\tSan Diego County\tH1\n92092\t6073\tLa jolla\tCA\tSan Diego County\tH1\n92182\t6073\tSan diego\tCA\tSan Diego County\tH1\n91948\t6073\tMount laguna\tCA\tSan Diego County\tH1\n92161\t6073\tSan diego\tCA\tSan Diego County\tH1\n94109\t6075\tSan francisco\tCA\tSan Francisco County\tH6\n94131\t6075\tSan francisco\tCA\tSan Francisco County\tH6\n94158\t6075\tSan francisco\tCA\tSan Francisco County\tH6\n94127\t6075\tSan francisco\tCA\tSan Francisco County\tH6\n94126\t6075\tSan francisco\tCA\tSan Francisco County\tH6\n94164\t6075\tSan francisco\tCA\tSan Francisco County\tH6\n94147\t6075\tSan francisco\tCA\tSan Francisco County\tH6\n94121\t6075\tSan francisco\tCA\tSan Francisco County\tH6\n94123\t6075\tSan francisco\tCA\tSan Francisco County\tH6\n94118\t6075\tSan francisco\tCA\tSan Francisco County\tH6\n94117\t6075\tSan francisco\tCA\tSan Francisco County\tH6\n94014\t6075\tDaly city\tCA\tSan Francisco County\tH6\n94188\t6075\tSan francisco\tCA\tSan Francisco County\tH6\n94159\t6075\tSan francisco\tCA\tSan Francisco County\tH6\n94110\t6075\tSan francisco\tCA\tSan Francisco County\tH6\n94129\t6075\tSan francisco\tCA\tSan Francisco County\tH6\n94141\t6075\tSan francisco\tCA\tSan Francisco County\tH6\n94107\t6075\tSan francisco\tCA\tSan Francisco County\tH6\n94124\t6075\tSan francisco\tCA\tSan Francisco County\tH6\n94134\t6075\tSan francisco\tCA\tSan Francisco County\tH6\n94103\t6075\tSan francisco\tCA\tSan Francisco County\tH6\n94104\t6075\tSan francisco\tCA\tSan Francisco County\tH6\n94105\t6075\tSan francisco\tCA\tSan Francisco County\tH6\n94112\t6075\tSan francisco\tCA\tSan Francisco County\tH6\n94122\t6075\tSan francisco\tCA\tSan Francisco County\tH6\n94133\t6075\tSan francisco\tCA\tSan Francisco County\tH6\n94132\t6075\tSan francisco\tCA\tSan Francisco County\tH6\n94143\t6075\tSan francisco\tCA\tSan Francisco County\tH6\n94140\t6075\tSan francisco\tCA\tSan Francisco County\tH6\n94108\t6075\tSan francisco\tCA\tSan Francisco County\tH6\n94116\t6075\tSan francisco\tCA\tSan Francisco County\tH6\n94102\t6075\tSan francisco\tCA\tSan Francisco County\tH6\n94111\t6075\tSan francisco\tCA\tSan Francisco County\tH6\n94114\t6075\tSan francisco\tCA\tSan Francisco County\tH6\n94115\t6075\tSan francisco\tCA\tSan Francisco County\tH6\n94130\t6075\tSan francisco\tCA\tSan Francisco County\tH6\n94119\t6075\tSan francisco\tCA\tSan Francisco County\tH6\n94146\t6075\tSan francisco\tCA\tSan Francisco County\tH6\n95202\t6077\tStockton\tCA\tSan Joaquin County\tH1\n95237\t6077\tLockeford\tCA\tSan Joaquin County\tH1\n95690\t6077\tWalnut grove\tCA\tSan Joaquin County\tH1\n95213\t6077\tStockton\tCA\tSan Joaquin County\tH1\n95208\t6077\tStockton\tCA\tSan Joaquin County\tH1\n95253\t6077\tVictor\tCA\tSan Joaquin County\tH1\n95211\t6077\tStockton\tCA\tSan Joaquin County\tH1\n95227\t6077\tClements\tCA\tSan Joaquin County\tH1\n95204\t6077\tStockton\tCA\tSan Joaquin County\tH1\n95205\t6077\tStockton\tCA\tSan Joaquin County\tH1\n95336\t6077\tManteca\tCA\tSan Joaquin County\tH1\n95366\t6077\tRipon\tCA\tSan Joaquin County\tH1\n95320\t6077\tEscalon\tCA\tSan Joaquin County\tH1\n95385\t6077\tVernalis\tCA\tSan Joaquin County\tH1\n95686\t6077\tThornton\tCA\tSan Joaquin County\tH1\n95240\t6077\tLodi\tCA\tSan Joaquin County\tH1\n95215\t6077\tStockton\tCA\tSan Joaquin County\tH1\n95210\t6077\tStockton\tCA\tSan Joaquin County\tH1\n95220\t6077\tAcampo\tCA\tSan Joaquin County\tH1\n95231\t6077\tFrench camp\tCA\tSan Joaquin County\tH1\n95209\t6077\tStockton\tCA\tSan Joaquin County\tH1\n95258\t6077\tWoodbridge\tCA\tSan Joaquin County\tH1\n95203\t6077\tStockton\tCA\tSan Joaquin County\tH1\n95206\t6077\tStockton\tCA\tSan Joaquin County\tH1\n95377\t6077\tTracy\tCA\tSan Joaquin County\tH1\n95269\t6077\tStockton\tCA\tSan Joaquin County\tH1\n95267\t6077\tStockton\tCA\tSan Joaquin County\tH1\n95207\t6077\tStockton\tCA\tSan Joaquin County\tH1\n95219\t6077\tStockton\tCA\tSan Joaquin County\tH1\n95632\t6077\tGalt\tCA\tSan Joaquin County\tH1\n95337\t6077\tManteca\tCA\tSan Joaquin County\tH1\n95330\t6077\tLathrop\tCA\tSan Joaquin County\tH1\n95241\t6077\tLodi\tCA\tSan Joaquin County\tH1\n95378\t6077\tTracy\tCA\tSan Joaquin County\tH1\n95236\t6077\tLinden\tCA\tSan Joaquin County\tH1\n95391\t6077\tTracy\tCA\tSan Joaquin County\tH1\n95304\t6077\tTracy\tCA\tSan Joaquin County\tH1\n95367\t6077\tRiverbank\tCA\tSan Joaquin County\tH1\n95376\t6077\tTracy\tCA\tSan Joaquin County\tH1\n95201\t6077\tStockton\tCA\tSan Joaquin County\tH1\n95234\t6077\tHolt\tCA\tSan Joaquin County\tH1\n95212\t6077\tStockton\tCA\tSan Joaquin County\tH1\n95242\t6077\tLodi\tCA\tSan Joaquin County\tH1\n95361\t6077\tOakdale\tCA\tSan Joaquin County\tH1\n95230\t6077\tFarmington\tCA\tSan Joaquin County\tH1\n93420\t6079\tArroyo grande\tCA\tSan Luis Obispo County\tH1\n93406
